vi "Test popup.vi"() -> ()   [LabVIEW 2017]
uses:
  Popup.lvclass
panel:
  in  "R2":u16(ring) items=["", "春", "夏", "秋", "冬"]
  in  "S1":string
  in  "R1":u16(ring) items=["", "数字", "下拉列表", "字符串", "下拉表"]
  in  "D0":i32
  in  "多列列表框":i32(listbox)
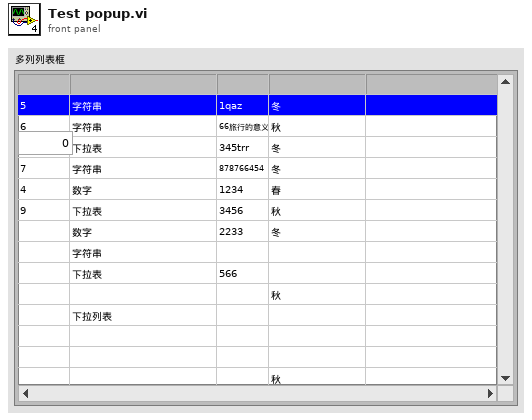
[diagram p1: front panel]
types:
  T1 = typedef "LVPoint32TypeDef.ctl" = cluster{"Horizontal":i32, "Vertical":i32}
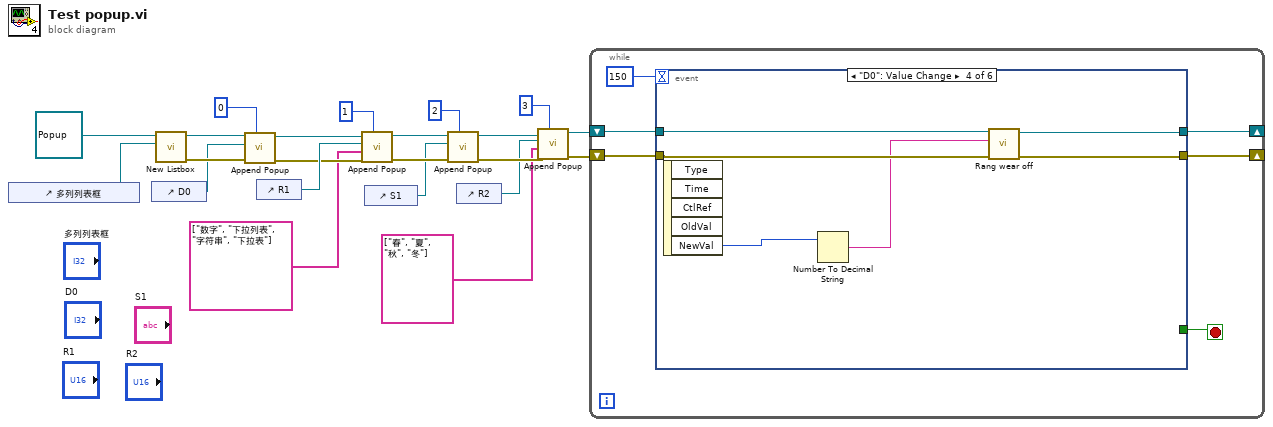
[diagram p0: block diagram]
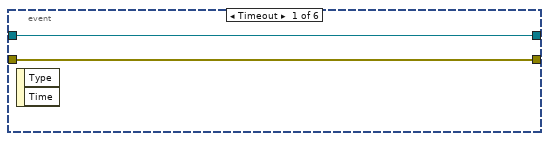
[diagram p2: hidden frame]
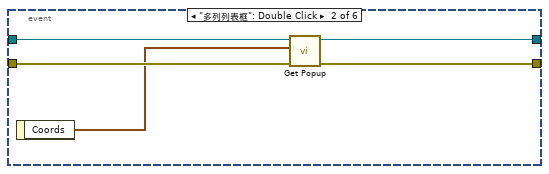
[diagram p3: hidden frame]
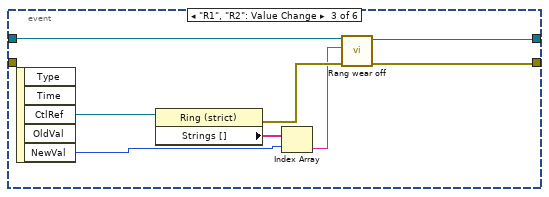
[diagram p4: hidden frame]
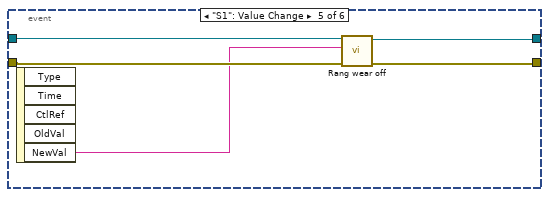
[diagram p5: hidden frame]
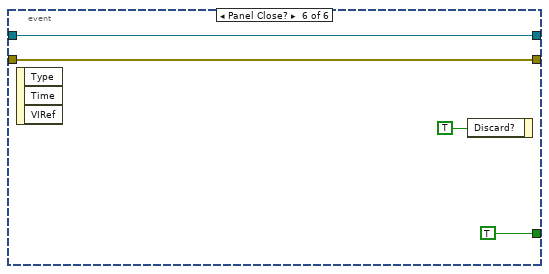
[diagram p6: hidden frame]
diagram:
  n1 = control-ref of="多列列表框"() -> (w21:refnum<vi>)
  n2 = control-ref of="D0"() -> (w17:refnum<vi>)
  n3 = call-dynamic "New Listbox.vi"("ListBox"=w21, "Popup 输入"=refnum<class "Popup.lvclass"> refnum) -> ("error out"=w18:errorcluster, "Popup 输出"=w20:refnum<class "Popup.lvclass">)  [unwired: 8 in]
  n4 = call-dynamic "Append Popup.vi"("Column"=0, "error in (no error)"=w18, "PopupRef"=w17, "Popup 输入"=w20) -> ("error out"=w13:errorcluster, "Popup 输出"=w16:refnum<class "Popup.lvclass">)  [unwired: 6 in]
  n5 = control-ref of="R1"() -> (w14:refnum<vi>)
  n6 = call-dynamic "Append Popup.vi"("Column"=1, "error in (no error)"=w13, "RangText"=string[] ["数字", "下拉列表", "字符串", "下拉表"], "PopupRef"=w14, "Popup 输入"=w16) -> ("error out"=w9:errorcluster, "Popup 输出"=w10:refnum<class "Popup.lvclass">)  [unwired: 5 in]
  n7 = control-ref of="S1"() -> (w8:refnum<vi>)
  n8 = call-dynamic "Append Popup.vi"("Column"=2, "error in (no error)"=w9, "PopupRef"=w8, "Popup 输入"=w10) -> ("error out"=w6:errorcluster, "Popup 输出"=w7:refnum<class "Popup.lvclass">)  [unwired: 6 in]
  n9 = control-ref of="R2"() -> (w2:refnum<vi>)
  n10 = call-dynamic "Append Popup.vi"("Column"=3, "error in (no error)"=w6, "RangText"=string[] ["春", "夏", "秋", "冬"], "PopupRef"=w2, "Popup 输入"=w7) -> ("error out"=w5:errorcluster, "Popup 输出"=w4:refnum<class "Popup.lvclass">)  [unwired: 5 in]
  n11 = while {
    shift-right: [w26] -> _
    shift-left: w5 -> [w28]
    shift-right: [w25] -> _
    shift-left: w4 -> [w24]
    stop <- w23 stop-if-true
    n12 = event shown="[3] \"D0\": Value Change" {
      selector: _ -> [_ _ _ _ _ _]
      dyn-events: _ -> [_ _ _ _ _ _]
      timeout: 150 -> [_ _ _ _ _ _]
      tunnel: w24 -> [w30 w35 w43 w49 w54 w56]
      tunnel: w28 -> [w29 w34 _ w45 w51 w55]
      tunnel: [w29 w32 w41 w47 w52 w55] -> w26
      tunnel: [w30 w31 w42 w48 w53 w56] -> w25
      tunnel: [_ _ _ _ _ TRUE] -> w23
      event Timeout {
        n13 = event-data() -> ()  [unwired: 1 in, 2 out]
      }
      event "多列列表框": Double Click {
        n14 = event-data() -> ("Coords"=w33:T1)  [unwired: 1 in]
        n15 = call "Get Popup.vi"("error in (no error)"=w34, "Point"=w33, "Popup 输入"=w35) -> ("error out"=w32:errorcluster, "Popup 输出"=w31:refnum<class "Popup.lvclass">)  [unwired: 7 in]
      }
      event "R1", "R2": Value Change {
        n16 = event-data() -> ("CtlRef"=w37:refnum<vi>, "NewVal"=w36:u16)  [unwired: 1 in, 3 out]
        n17 = property class="Ring (strict)"(reference=w37) -> (error out=w40:errorcluster, "Strings []"=w39:string[])  [unwired: 1 in, 1 out]
        n18 = Index Array(array=w39, index=w36) -> (element=w38:string)
        n19 = call-dynamic "Rang wear off.vi"("error in (no error)"=w40, "字符串"=w38, "Popup 输入"=w43) -> ("error out"=w41:errorcluster, "Popup 输出"=w42:refnum<class "Popup.lvclass">)  [unwired: 7 in]
      }
      event "D0": Value Change {
        n20 = event-data() -> ("NewVal"=w46:i32)  [unwired: 1 in, 4 out]
        n21 = Number To Decimal String(number=w46) -> (decimal integer string=w44:string)  [unwired: 1 in]
        n22 = call-dynamic "Rang wear off.vi"("error in (no error)"=w45, "字符串"=w44, "Popup 输入"=w49) -> ("error out"=w47:errorcluster, "Popup 输出"=w48:refnum<class "Popup.lvclass">)  [unwired: 7 in]
      }
      event "S1": Value Change {
        n23 = event-data() -> ("NewVal"=w50:string)  [unwired: 1 in, 4 out]
        n24 = call-dynamic "Rang wear off.vi"("error in (no error)"=w51, "字符串"=w50, "Popup 输入"=w54) -> ("error out"=w52:errorcluster, "Popup 输出"=w53:refnum<class "Popup.lvclass">)  [unwired: 7 in]
      }
      event Panel Close? {
        n25 = event-data() -> ()  [unwired: 1 in, 3 out]
        n26 = event-data("Discard?"=TRUE) -> ()  [unwired: 1 in, 1 out]
      }
    }
  }
